vi "Byte to Bits.vi"(0 "Byte":u8 format="%02x", 7 "Bit Width":i32=8, 11 "error in (no error)":errorcluster) -> (4 "Bits":u8[](array[numeric]), 15 "error out":errorcluster)   [LabVIEW 2018, in "MIPI RFFE API.lvlib"]
uses:
  MIPI RFFE API.lvlib
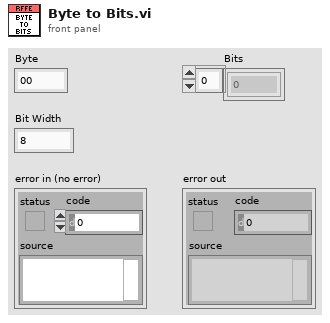
[diagram p1: front panel]
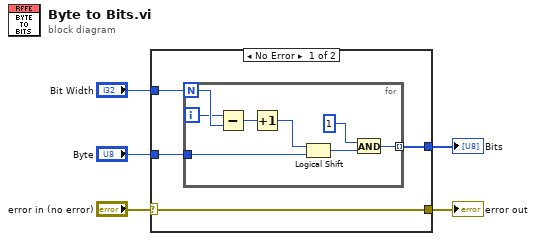
[diagram p0: block diagram]
diagram:
  n1 = case shown="No Error" "error in (no error)" {
    selector: "error in (no error)" -> [w9 w18]
    tunnel: [w9 w18] -> w4
    tunnel: "Byte" -> [w7 _]
    tunnel: "Bit Width" -> [w8 _]
    tunnel: [w6 _] -> w1
    frame No Error {
      n2 = for {
        N: w8 -> [w17]
        tunnel: w7 -> [w13]
        tunnel: [w10] -> w6 mode=indexing
        i -> [w16]
        n3 = Subtract(x=w16, y=w17) -> (x-y=w15:i32)
        n4 = Increment(x=w15) -> (x+1=w14:i32)
        n5 = Logical Shift(y=w14, x=w13) -> (x << y=w12:u8)
        n6 = And(x=u8 1, y=w12) -> (x .and. y?=w10:u8)
      }
    }
    frame Error {
    }
  }
  "error out" <- w4
  "Bits" <- w1
